vi "Read Discrete Inputs.vi"(8 "error in":errorcluster, 9 "number of inputs":u16, 10 "starting address":u16, 11 "Modbus instance in":refnum<class "Modbus API.lvclass">) -> (0 "error out":errorcluster, 2 "discrete inputs":bool[](array[boolean]), 3 "Modbus instance out":refnum<class "Modbus API.lvclass">)   [LabVIEW 2012, in "Modbus API.lvclass"]
doc: "Reads <B>number of inputs</B> discrete inputs starting at <B>starting address</B> from the device."
uses:
  Modbus API.lvclass
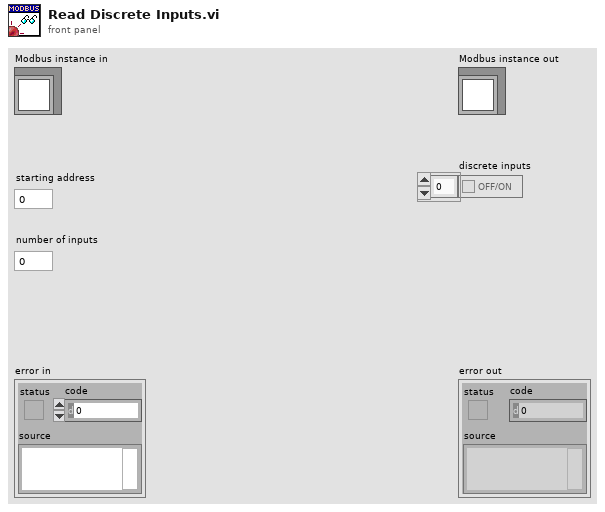
[diagram p1: front panel]
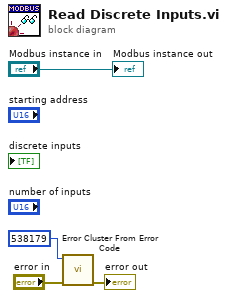
[diagram p0: block diagram]
diagram:
  n1 = call <vilib>:"Error Cluster From Error Code.vi"("error in (no error)"="error in", "error code (0)"=538179) -> ("error out"=→"error out":errorcluster)  [unwired: 7 in]
  "Modbus instance out" <- "Modbus instance in"
